vi "Read 1D Array I64.vi"(8 "error in (no error)":errorcluster, 9 "start index (0)":i64, 10 "number of elements":i64, 11 "pointer in":u64) -> (0 "error out":errorcluster, 1 "start index out":i64, 2 "value":i64[](array[numeric]), 3 "pointer out":u64)   [LabVIEW 2016, in "Linux RT IPC.Shared Memory.lvlib"]
uses:
  Linux RT IPC.Shared Memory.lvlib
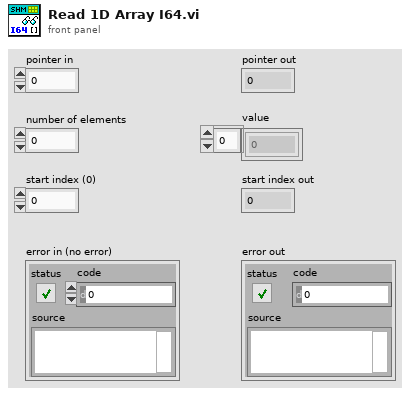
[diagram p1: front panel]
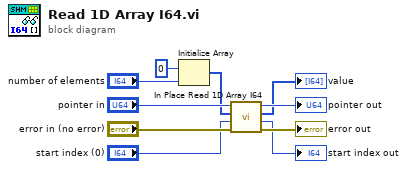
[diagram p0: block diagram]
diagram:
  n1 = Initialize Array(i64 0, "number of elements") -> (w4:i64[])
  n2 = call "In Place Read 1D Array I64.vi"("error in (no error)"="error in (no error)", "start index (0)"="start index (0)", "values in"=w4, "pointer in"="pointer in") -> ("error out"=→"error out":errorcluster, "start index out"=→"start index out":i64, "values out"=→"value":i64[], "pointer out"=→"pointer out":u64)  [unwired: 4 in]
